vi "Parse IPG Temperature.vi"(11 "Thermistor Data":string="ThermBias=1468\r\nThermInput=1079\r\nThermOffset=590") -> (1 "Resistance (ohms)":dbl=nan format="%.3f", 3 "Temperature C":dbl=nan format="%.3f")   [LabVIEW 2010]
doc: "This function parses an IPG Thermistor Status string and converts it to a temperature in degrees Celsius.\n\nIf the status string format is incorrect, NaN values will be returned."
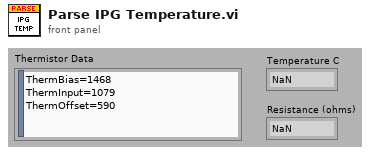
[diagram p1: front panel]
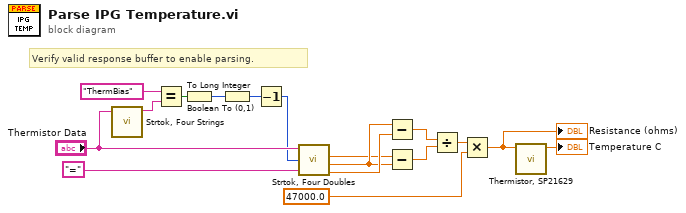
[diagram p0: block diagram]
diagram:
  # "Verify valid response buffer to enable parsing."
  n1 = call "Strtok, Four Strings.vi"("input string"="Thermistor Data") -> ("token 1"=w16:string)  [unwired: 2 in, 3 out]
  n2 = Equal?(x="ThermBias", y=w16) -> (x = y?=w13:bool)
  n3 = Boolean To (0,1)(Boolean=w13) -> (0, 1=w11:i16)
  n4 = To Long Integer(number=w11) -> (32bit integer=w10:i32)
  n5 = Decrement(x=w10) -> (x-1=w12:i32)
  n6 = call "Strtok, Four Doubles.vi"("delimiters (\\s\\t\\r\\n=)"="=" ("delimiters (\\s\\t\\r\\n=)"), "offset"=w12, "input string"="Thermistor Data") -> ("x4"=w7:dbl, "x3"=w6:dbl, "x 2"=w5:dbl)  [unwired: 1 out]
  n7 = Subtract(x=w6, y=w7) -> (x-y=w2:dbl)
  n8 = Subtract(x=w5, y=w6) -> (x-y=w3:dbl)
  n9 = Divide(x=w2, y=w3) -> (x/y=w8:dbl)
  n10 = Multiply(x=w8, y=47000.0) -> (x*y=w1:dbl)
  "Resistance (ohms)" <- w1
  n11 = call "Thermistor, SP21629.vi"("resistance (ohms)"=w1) -> ("temperature (C)"=→"Temperature C":dbl)  [unwired: 9 in, 1 out]
